vi "Produced Versions.vi"(8 "error in":errorcluster, 9 "Produced Method":u16(ring) items=["Box", "EtFlocSedFi", "LFOM", "Tank"], 11 "Version Ref":refnum<vi>) -> (0 "error out":errorcluster, 3 "Designs in Method version":path)   [LabVIEW 2011]
uses:
  Folders.ctl
  Design Server.lvlib
panel:
  out "Produced Versions":string[](array[string])
  out "Produced Methods":string[](array[string])
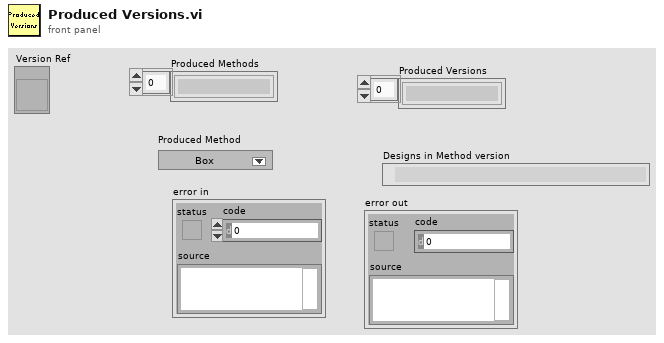
[diagram p1: front panel]
types:
  T1 = typedef "Design Server.lvlib/Folders.ctl" = enum16{"MathcadMethods", "RequestedDesigns", "CompletedDesigns", "MathcadCode", "CollabnetSVN.exe"}
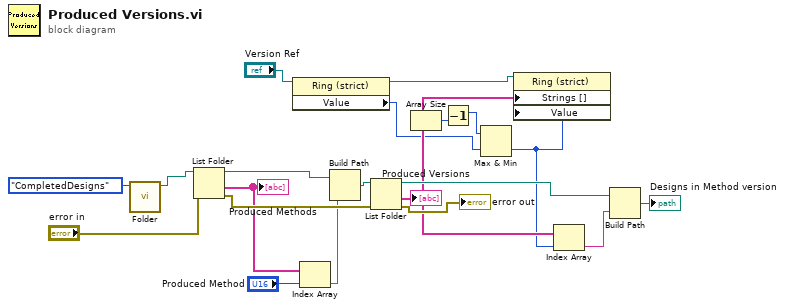
[diagram p0: block diagram]
diagram:
  n1 = call "Folder.vi"("Folders"=Folders."CompletedDesigns") -> ("FolderPath"=w19:path)  [unwired: 8 in, 2 out]
  n2 = List Folder(path=w19, error in="error in") -> (path out=w12:path, folder names=w15:string[], error out=w16:errorcluster)  [unwired: 2 in, 1 out]
  "Produced Methods" <- w15
  n3 = property class="Ring (strict)"(reference="Version Ref") -> (reference out=w2:refnum<vi>, "Value"=w1:u16)  [unwired: 1 in, 1 out]
  n4 = Index Array(array=w15, index="Produced Method") -> (element=w13:string)
  n5 = Build Path(base path=w12, name or relative path=w13) -> (appended path=w17:path)
  n6 = List Folder(path=w17, error in=w16) -> (path out=w8:path, folder names=w6:string[], error out=→"error out":errorcluster)  [unwired: 2 in, 1 out]
  "Produced Versions" <- w6
  n7 = Array Size(array=w6) -> (size(s)=w10:i32)
  n8 = Decrement(x=w10) -> (x-1=w9:i32)
  n9 = Max & Min(x=w9, y=w1) -> (min(x,y)=w5:i32)  [unwired: 1 out]
  n10 = property class="Ring (strict)"(reference=w2, "Strings []"=w6, "Value"=w5) -> ()  [unwired: 1 in, 2 out]
  n11 = Index Array(array=w6, index=w5) -> (element=w7:string)
  n12 = Build Path(base path=w8, name or relative path=w7) -> (appended path=→"Designs in Method version":path)
